vi "Read Panel Data.vi"(8 "Error In":errorcluster, 10 "Field":string, 11 "Panel Helper in":refnum<class "Panel Helper.lvclass">) -> (0 "Error Out":errorcluster, 2 "Found?":bool, 3 "Panel Data":variant)   [LabVIEW 2020, in "Panel.lvlib" / "Panel Helper.lvclass"]
doc: "Reads a field from the Panel Data\n\n<B>Panel Helper In:</B> Panel Helper object to write panel data\n<B>Field:</B> Data field associated with the panel data.\n<B>Error In:</B> Describes error conditions that occur before this node runs.\n\n<B>Panel Data:</B> Panel data associated with the field.\n<B>Found?:</B> Indicates if the Panel Data was found.\n<B>Error Out:</B> Contains error information.\n\n----\nPlease see the following web address for additional documentation and tutorial information:\nhttp://www.mooregoodideas.com/mgi-panel-manager/\n\nAuthor: Derek Trepanier\n\nCopyright (c) 2018, Moore Good Ideas, Inc.\n\nAll rights reserved.\n\nRedistribution and use in source and binary forms, with or without modification, are permitted provided that the following conditions are met:\n\n * Redistributions of source code must retain the above copyright notice, this list of conditions and the following disclaimer.\n * Redistributions in binary form must reproduce the above copyright notice, this list of conditions and the following disclaimer in the documentation and/or other materials provided with the distribution.\n * Neither the name of Moore Good Ideas, Inc. nor the names of its contributors may be used to endorse or promote products derived from this software without specific prior written permission.\n\nTHIS SOFTWARE IS PROVIDED BY THE COPYRIGHT HOLDERS AND CONTRIBUTORS \"AS IS\" AND ANY EXPRESS OR IMPLIED WARRANTIES, INCLUDING, BUT NOT LIMITED TO, THE IMPLIED WARRANTIES OF MERCHANTABILITY AND FITNESS FOR A PARTICULAR PURPOSE ARE DISCLAIMED. IN NO EVENT SHALL THE COPYRIGHT OWNER OR CONTRIBUTORS BE LIABLE FOR ANY DIRECT, INDIRECT, INCIDENTAL, SPECIAL, EXEMPLARY, OR CONSEQUENTIAL DAMAGES (INCLUDING, BUT NOT LIMITED TO, PROCUREMENT OF SUBSTITUTE GOODS OR SERVICES; LOSS OF USE, DATA, OR PROFITS; OR BUSINESS INTERRUPTION) HOWEVER CAUSED AND ON ANY THEORY OF LIABILITY, WHETHER IN CONTRACT, STRICT LIABILITY, OR TORT (INCLUDING NEGLIGENCE OR OTHERWISE) ARISING IN ANY WAY OUT OF THE USE OF THIS SOFTWARE, EVEN IF ADVISED OF THE POSSIBILITY OF SUCH DAMAGE."
uses:
  <vilib>/MGI/Panel Manager/Panel/Panel Helper/Panel Helper.lvclass
  <vilib>/MGI/Panel Manager/Panel/Panel Helper/Panel Helper.lvclass/Panel Helper.ctl
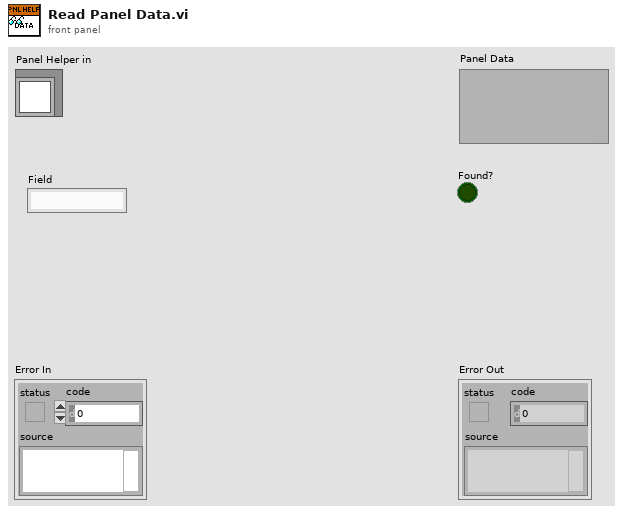
[diagram p1: front panel]
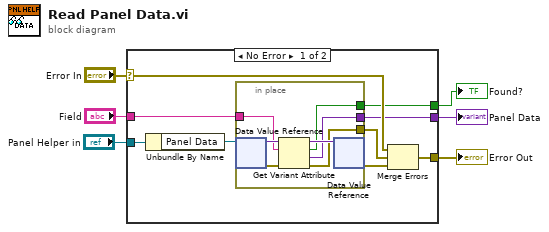
[diagram p0: block diagram]
diagram:
  n1 = case shown="No Error" "Error In" {
    selector: "Error In" -> [w15 w23]
    tunnel: [w10 w23] -> w5
    tunnel: "Panel Helper in" -> [w14 _]
    tunnel: "Field" -> [w12 _]
    tunnel: [w11 _] -> w2
    tunnel: [w7 _] -> w1
    frame No Error {
      n2 = Unbundle By Name(w14) -> ("Panel Data"=w13:refnum<data-value>)
      n3 = in-place {
        in-place-border: w12 -> [w20]
        in-place-border: [w19] -> w11
        in-place-border: [w17] -> w9
        in-place-border: [w16] -> w7
        n4 = in-place-dvr #1(w13) -> (w22:variant, w18:errorcluster)
        n5 = Get Variant Attribute(Variant=w22, name=w20, error in=w18) -> (duplicate Variant=w21:variant, found=w16:bool, value=w19:variant, error out=w17:errorcluster)  [unwired: 1 in]
        n6 = in-place-dvr #1(w21) -> (w8:errorcluster)  [unwired: 1 out]
      }
      n7 = Merge Errors(w15, w9, w8) -> (w10:errorcluster)
    }
    frame Error {
    }
  }
  "Error Out" <- w5
  "Panel Data" <- w2
  "Found?" <- w1
